vi "Swerve Drive Controller.vi"(8 "error in":errorcluster) -> ()   [LabVIEW 2015]
doc: "This VI executes continuously carrying out the current operation and responding to updates or new operations. It will often contain the timing or control code that is difficult to place directly in TeleOp. This VI generally opens all sensors and motors and isolates the rest of the robot code from knowing how the operations are carried out."
uses:
  Swerve Drive Setpoints.ctl
  Swerve Drive Operations.ctl
  <vilib>/Rock Robotics/WPI/CAN/TalonSRX/WPI_CANTalonSRX_APIControlMode.ctl
  Support Code/Team900-VIs/Team900SwerveDrive/SwerveDriveFuse.vi
  Swerve Drive Published Globals.vi
  <vilib>/Rock Robotics/Network Tables/SD Read Boolean.vi
  <vilib>/Rock Robotics/Network Tables/NT Read Numeric Array.vi
  Support Code/Team900-VIs/Team900SwerveDrive/SwerveGlobalData.vi
  Support Code/Team900-VIs/Team900SwerveDrive/Team900SwerveDrive.lvlib
  Support Code/Team900-VIs/navX Library v2/navX Library v2.lvlib
panel:
  out "Speed Chart":cluster{dbl, "Encoder Velocity":dbl}[](graph)
  out "Position Chart":cluster{dbl, "Encoder Velocity":dbl}[](graph)
  out "Current\nCmd":string
  # "Tip: It may be helpful to observe inputs and sensor values.\nYou may also want to display tuning or debugging controls."
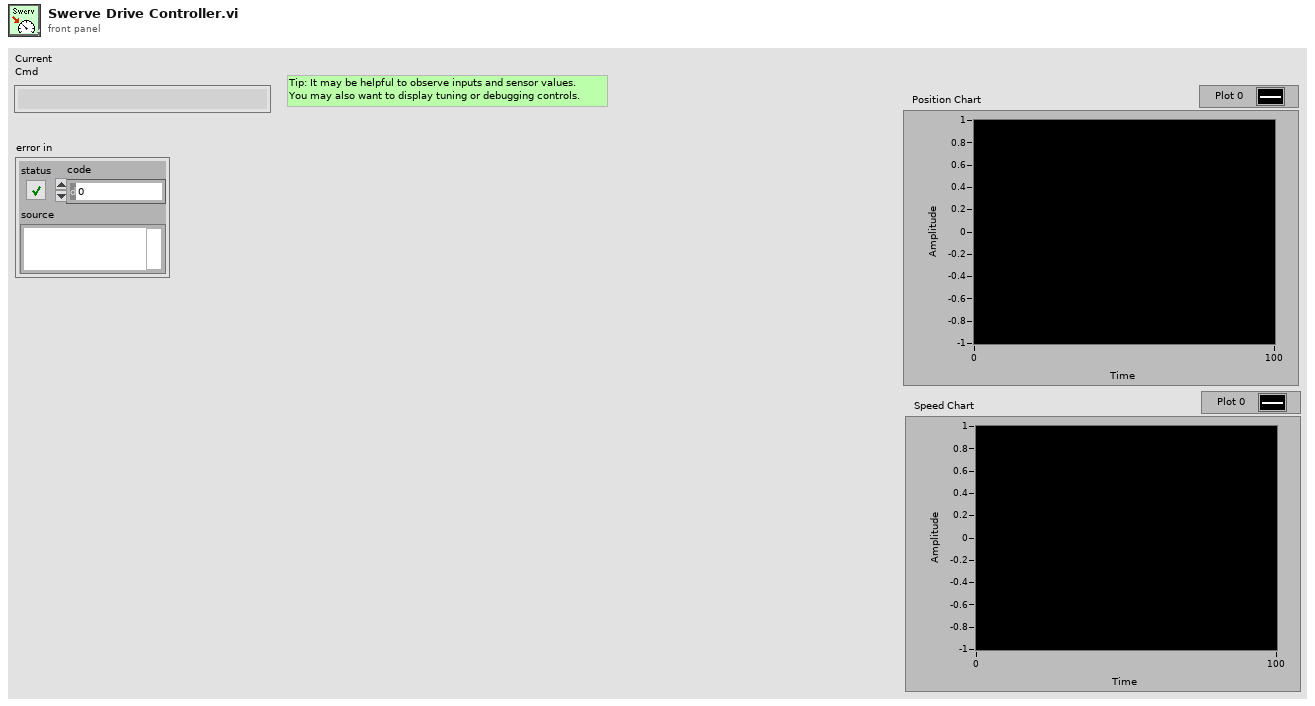
[diagram p1: front panel]
types:
  T1 = typedef "Swerve Drive Setpoints.ctl" = cluster{"Operation":T2, "Duration":dbl, "Strafe Joystick Axes":cluster{"X":dbl, "Y":dbl}, "Face Joystick Axes":cluster{"X":dbl, "Y":dbl}, "Trigger Axes":cluster{"Left":dbl, "Right":dbl}, "Coordinates":cluster{"X":dbl, "Y":dbl, "Angle":dbl}}
  T2 = typedef "Swerve Drive Operations.ctl" = enum16{"Reserve", "Read Current", "Immediate", "Go to Coordinate", "Drive Immediate (Turn Speed/Face and Stafe)"}
  T3 = typedef "Command Status Info.ctl" = cluster{"Name":string, "Status":T4, "notifier out":T5}
  T4 = typedef "Completion Status.ctl" = enum16{"Successful", "Aborted", "Incomplete"}
  T5 = typedef "Completion Notifier.ctl" = refnum<notifier>
  T6 = cluster{"Default Command":T1, "Command Timing":cluster{"Start Time (ms)":u32, "Iterations":i32}, "Command Arguments":cluster{"Command Info":T3, "Description":string, "Default Command":T1, "notifier out":refnum<notifier>, "Subsystem Name":string}}
  T7 = typedef "navX Library v2.lvlib/Z900_navX_DeviceTypeDef.ctl" = cluster{"Interface":cluster{"Protocol":T8, "Update Rate (4Hz-60Hz)":u8, "navX Open TypeDef":variant}, "Notify Packet":refnum<notifier>, "Loop VI Refnum":refnum<vi>, "Ready to Close Occurrence Refnum":refnum<k4>}
  T8 = typedef "navX Library v2.lvlib/Z900_navX_ProtocolTypeDef.ctl" = enum16{"SERIAL", "I2C", "SPI"}
  T9 = typedef "WPI_MotorControlDeviceRef.ctl" = cluster{"DeviceStatus":errorcluster, "Type":T10, "PWM":cluster{"PWM Channel":T11, "DeadBand":T12}, "CAN":cluster{"Device Number":u8, "Control Mode":T13, "Semaphore":T14, "Max Vout":dbl, "TalonSRX Control Mode":T15}, "Invert":bool}
  T10 = typedef "WPI_MotorControlType.ctl" = enum16{"PWM", "CAN", "CANTalonSRX"}
  T11 = typedef "FPGA_DIOPWMChannel.ctl" = enum8{"PWM 0", "PWM 1", "PWM 2", "PWM 3", "PWM 4", "PWM 5", "PWM 6", "PWM 7", "PWM 8", "PWM 9", "PWM MXP 0", "PWM MXP 1", "PWM MXP 2", "PWM MXP 3", "PWM MXP 4", "PWM MXP 5", "PWM MXP 6", "PWM MXP 7", "PWM MXP 8", "PWM MXP 9", "Invalid"}
  T12 = typedef "WPI_PWMDeadband.ctl" = cluster{"Name":string, "maxPositivePwm":i32, "minPositivePwm":i32, "centerPwm":i32, "maxNegativePwm":i32, "minNegativePwm":i32, "angularRange":u16}
  T13 = typedef "WPI_CANJaguar_ControlMode.ctl" = enum8{"Percent VBus", "Current", "Speed", "Position", "Voltage"}
  T14 = typedef "Semaphore RefNum" = refnum<k1>
  T15 = typedef "WPI_CANTalonSRX_APIControlMode.ctl" = enum8{"Percent VBus", "Speed", "Position", "Slave", "Unchanged / Invalid", "Voltage Compensation", "Current", "Motion Profile"}
  T16 = cluster{"Yaw":dbl, "Roll":dbl, "Pitch":dbl, "Heading":dbl, "Fused Heading":dbl}
  T17 = cluster{"Steering Motor Refs[0]":T9, "Steering Motor Refs[1]":T9, "Steering Motor Refs[2]":T9, "Steering Motor Refs[3]":T9}
  T18 = typedef "WPI_CANTalonSRX_GlobalStatus.ctl" = cluster{"Applied Throttle":dbl, "Module Enabled":bool, "CAN Error":errorcluster, "Closed Loop Error":dbl, "Forward Limit Switch Closed":bool, "Reverse Limit Switch Closed":bool, "Sensor Position":dbl, "Sensor Velocity":dbl, "Current":dbl, "Sticky Fault - Over Temp":bool, "Sticky Fault - Under Voltage":bool, "Sticky Fault - Forward Limit":bool, "Sticky Fault - Reverse Limit":bool, "Sticky Fault - Forward Soft Limit":bool, "Sticky Fault - Reverse Soft Limit":bool, "Brake is Enabled":bool, "Encoder Position":dbl, "Encoder Velocity":dbl, "Encoder Index Count":dbl, "Encoder A Pin State":bool, "Encoder B Pin State":bool, "Encoder Index Pin State":bool, "Analog In":dbl, "Analog In Velocity":dbl, "Temperature (C)":dbl, "Battery Voltage":dbl, "Control 5 Is Supported":bool, "Current Profile Slot Select":dbl, "Pos Div 8":bool, "Vel Div 4":bool, "Pulse Width Position":i32, "Pulse Width Velocity":i32, "Pulse Width Rise To Rise (us)":i32, "Pulse Width Rise To Fall (us)":i32, "Mot Prof Active Is Under Run":bool, "Mot Prof Active Has Under Run":bool, "Mot Prof Active Is Last":bool, "Mot Prof Active Velocity Only":bool, "Mot Prof Active Is Valid":bool, "Mot Prof Buffer Is Full":bool, "Mot Prof Active Profile Slot Select":i32, "Mot Prof NextID":i32, "Mot Prof Count":i32, "Mot Prof Active Velocity":dbl, "Mot Prof Active Position":dbl, "Mot Prof Output Enable":i32}
  T19 = cluster{"output angle":dbl, "Encoder Velocity":dbl}
  T20 = cluster{"[0]":dbl, "[1]":dbl, "[2]":dbl, "[3]":dbl}
  T21 = cluster{"Numeric Array[0]":dbl, "Numeric Array[1]":dbl, "Numeric Array[2]":dbl}
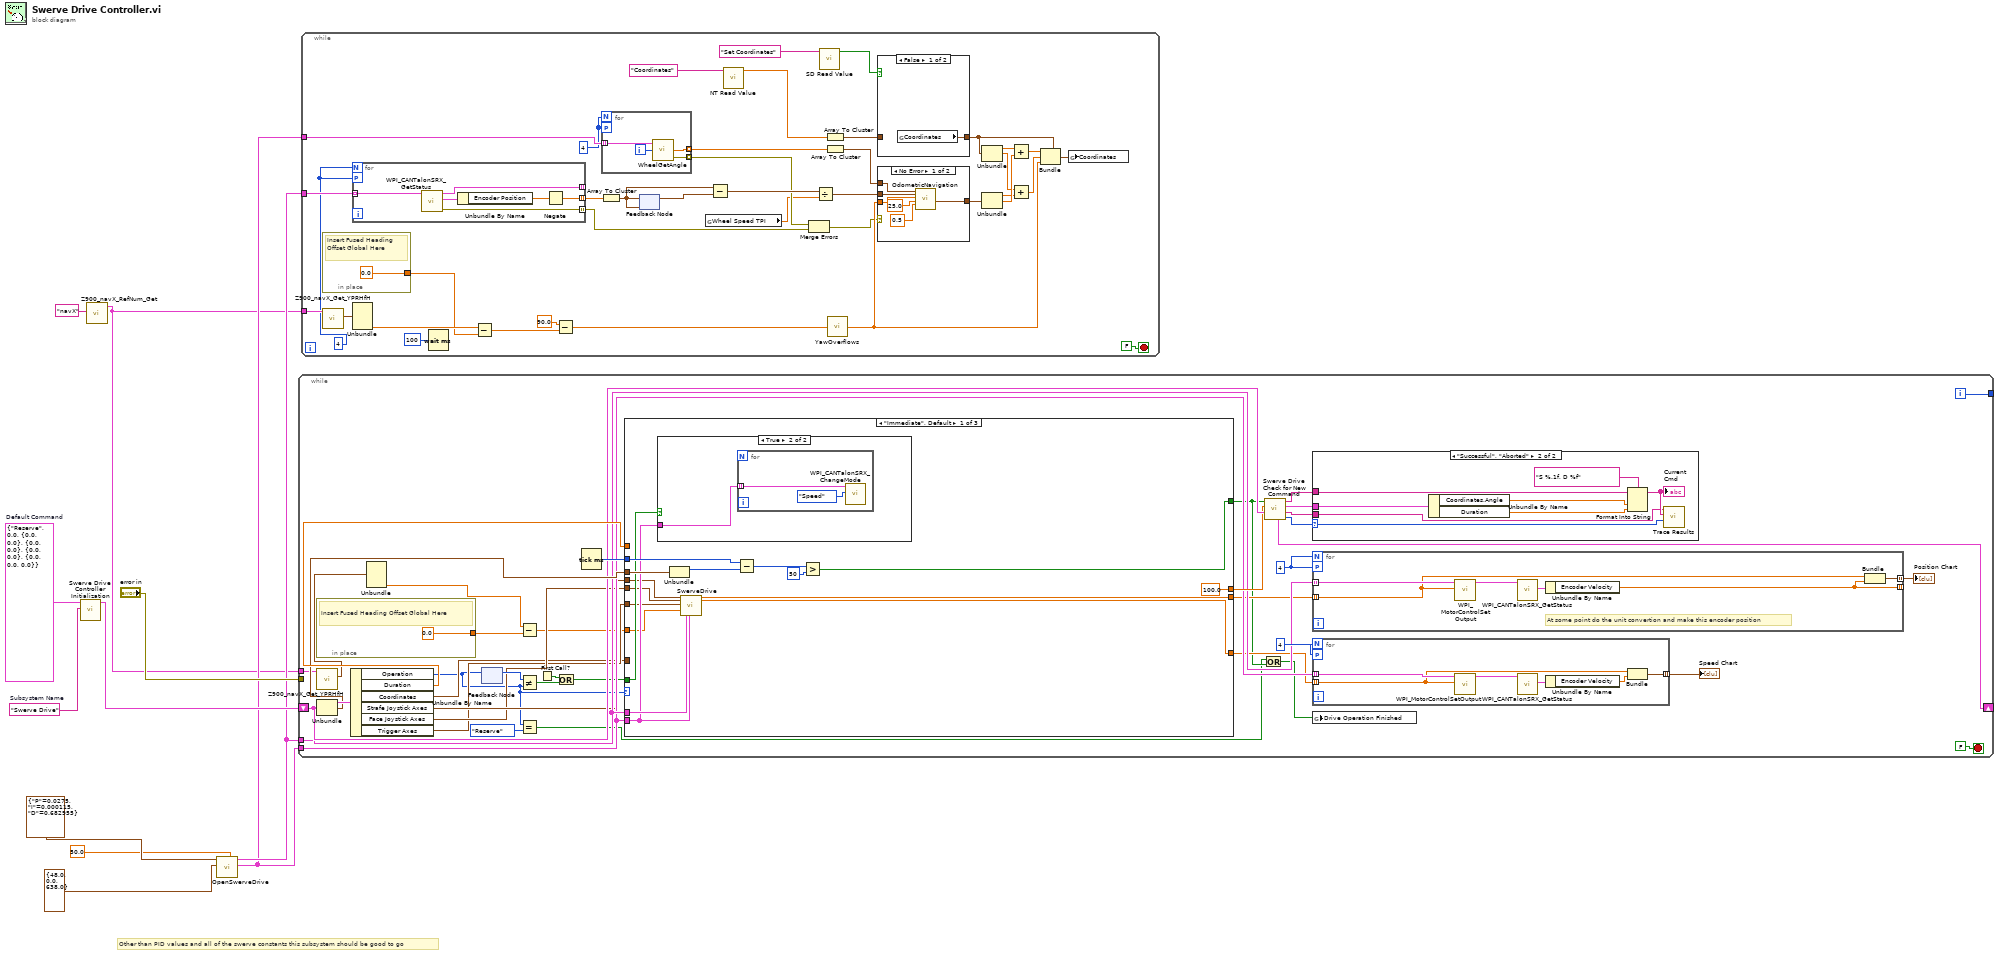
[diagram p0: block diagram]
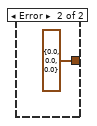
[diagram p2: hidden frame]
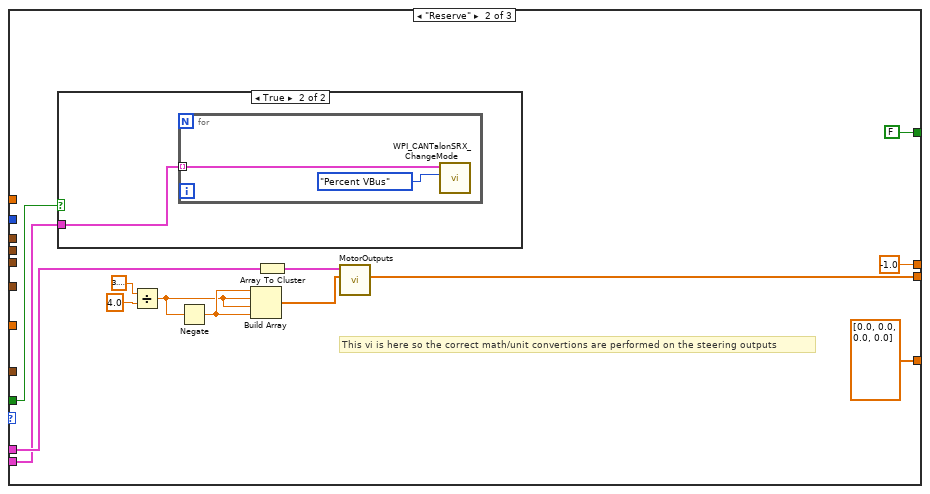
[diagram p6: hidden frame]
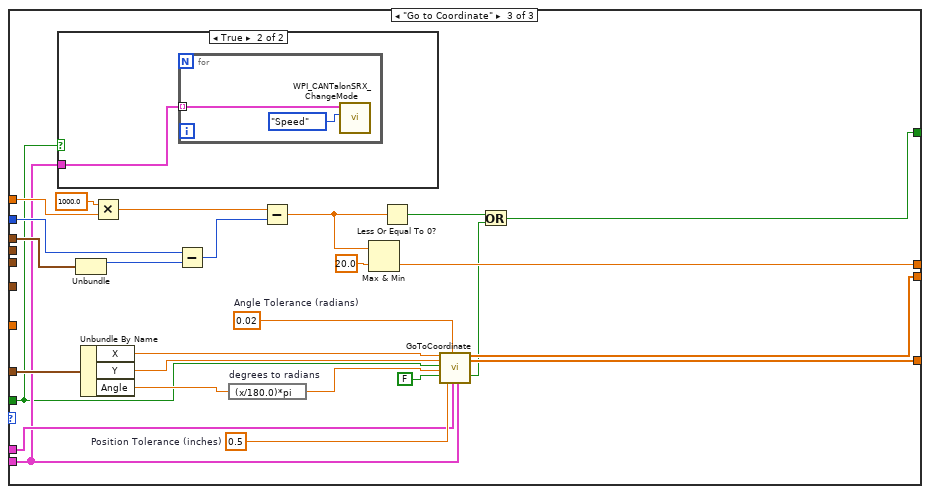
[diagram p8: hidden frame]
diagram:
  w8 = T1 {"Operation"=enum."Reserve", "Duration"=0.0, "Strafe Joystick Axes"={"X"=0.0, "Y"=0.0}, "Face Joystick Axes"={"X"=0.0, "Y"=0.0}, "Trigger Axes"={"Left"=0.0, "Right"=0.0}, "Coordinates"={"X"=0.0, "Y"=0.0, "Angle"=0.0}}  # Default Command
  w9 = "Swerve Drive"  # Subsystem Name
  # "Other than PID values and all of the swerve constants this subsystem should be good to go"
  n1 = call "Swerve Drive Controller Initialization.vi"("Subsystem Name"=w9, "Default Command"=w8) -> ("Command Info"=w10:T6)  [unwired: 9 in]
  n2 = call "Z900_navX_RefNum_Get.vi"("refnum name"="navX") -> ("navX Device"=w1:T7)  [unwired: 9 in, 1 out]
  n3 = call "OpenSwerveDrive.vi"("Ramp Rate"=50.0, "Speed PID"=cluster{"P":dbl, "I":dbl, "D":dbl} {"P"=48.0, "I"=0.0, "D"=638.0}, "Steering PID"=cluster{"P":dbl, "I":dbl, "D":dbl} {"P"=0.0275, "I"=0.000115, "D"=0.682955}) -> ("Speed Motor Refs"=w2:T9[], "Steering Motor Refs"=w3:T9[])  [unwired: 4 in, 1 out]
  n4 = while {
    shift-right: [w43] -> _
    shift-left: w10 -> [w44]
    tunnel: [w49] -> _
    tunnel: "error in" -> [_]
    tunnel: w3 -> [w33]
    tunnel: w2 -> [w32]
    tunnel: w1 -> [w13]
    i -> [w49]
    stop <- FALSE stop-if-true
    w34 = 4
    w35 = 4
    n5 = in-place {
      in-place-border: [0.0] -> w14
      # "Insert Fused Heading Offset Global Here"
    }
    n6 = call "Z900_navX_Get_YPRHfH.vi"("navX Device"=w13) -> ("YRPHfH"=w16:T16)  [unwired: 7 in, 3 out]
    n7 = Unbundle(w44) -> ("Default Command"=w48:T1, "Command Timing"=w45:cluster{"Start Time (ms)":u32, "Iterations":i32})  [unwired: 1 out]
    n8 = Unbundle By Name(w48) -> ("Operation"=w19:T2, "Duration"=w47:dbl, "Coordinates"=w22:cluster{"X":dbl, "Y":dbl, "Angle":dbl}, "Strafe Joystick Axes"=w25:cluster{"X":dbl, "Y":dbl}, "Face Joystick Axes"=w24:cluster{"X":dbl, "Y":dbl}, "Trigger Axes"=w23:cluster{"Left":dbl, "Right":dbl})
    n9 = Unbundle(w16) -> ("Fused Heading"=w15:dbl)  [unwired: 4 out]
    n10 = feedback-in #1(w19) -> ()
    n11 = feedback #1() -> (w29:T2)  [unwired: 1 in]
    n12 = Subtract(x=w15, y=w14) -> (x-y=w12:dbl)
    n13 = Not Equal?(x=w29, y=w19) -> (x != y?=w28:bool)
    n14 = Equal?(x=w19, y=Swerve_Drive_Operations."Reserve") -> (x = y?=w17:bool)
    n15 = First Call?() -> (First Call?: T/F=w27:bool)
    n16 = Or(x=w27, y=w28) -> (x .or. y?=w26:bool)
    n17 = Tick Count (ms)() -> (millisecond timer value=w46:u32)
    n18 = case shown="\"Immediate\", Default" w19 {
      tunnel: [100.0 -1.0 w121] -> w42
      tunnel: [w81 FALSE ("ignore previous (F)") w124] -> w21
      tunnel: w45 -> [w83 _ w132]
      tunnel: w47 -> [_ _ w129]
      tunnel: w46 -> [w82 _ w130]
      tunnel: w33 -> [w80 w94 w113]
      tunnel: w32 -> [w76 w91 w108]
      tunnel: [w79 w95 w111] -> w31
      tunnel: [w78 dbl[] [0.0, 0.0, 0.0, 0.0] ("appended array") w112] -> w30
      tunnel: w26 -> [w77 w92 w107]
      tunnel: w25 -> [w75 _ _]
      tunnel: w24 -> [w74 _ _]
      tunnel: w23 -> [w73 _ _]
      tunnel: w22 -> [_ _ w120]
      tunnel: w12 -> [w72 _ _]
      frame "Immediate", Default {
        n19 = case shown="True" w77 {
          tunnel: w76 -> [_ w88]
          frame False {
          }
          frame True {
            n20 = for {
              tunnel: w88 -> [w90] mode=indexing
              n21 = call <vilib>:"WPI_CANTalonSRX_ChangeMode.vi"("Control Mode"=WPI_CANTalonSRX_APIControlMode."Speed", "CAN Talon SRX Ref"=w90) -> ()  [unwired: 8 in, 2 out]
            }
          }
        }
        n22 = Unbundle(w83) -> ("Start Time (ms)"=w86:u32)  [unwired: 1 out]
        n23 = call-poly "SwerveDrive.vi"("Strafe Joystick Axes"=w75, "Face Joystick Axes"=w74, "Trigger Axes"=w73, "Angle (degrees; 0 = right)"=w72, "Steering Motor Refs"=w80, "Speed Motor Refs"=w76) -> ("Steering Motor Setpoints"=w79:dbl[], "Speed Motor Setpoints"=w78:dbl[])  [unwired: 10 in, 2 out]
        n24 = Subtract(x=w82, y=w86) -> (x-y=w85:u32)
        n25 = Greater?(x=w85, y=u8 50 ("Left Motor")) -> (0:w81:bool)
      }
      frame "Reserve" {
        # "This vi is here so the correct math/unit convertions are performed on the steering outputs"
        n26 = case shown="True" w92 {
          tunnel: w91 -> [_ w104]
          frame False {
          }
          frame True {
            n27 = for {
              tunnel: w104 -> [w106] mode=indexing
              n28 = call <vilib>:"WPI_CANTalonSRX_ChangeMode.vi"("Control Mode"=WPI_CANTalonSRX_APIControlMode."Percent VBus", "CAN Talon SRX Ref"=w106) -> ()  [unwired: 8 in, 2 out]
            }
          }
        }
        n29 = Divide(x=3.141592653589793, y=4.0) -> (x/y=w100:dbl)
        n30 = Negate(x=w100) -> (-x=w101:dbl)
        n31 = Build Array(w101, w100, w100, w101) -> (w97:dbl[])
        n32 = Array To Cluster(array=w94) -> (cluster=w93:T17)
        n33 = call "MotorOutputs.vi"("Target Angles"=w97, "Steering Refnums In"=w93) -> ("Steering Motor Setpoints"=w95:dbl[])  [unwired: 6 in, 3 out]
      }
      frame "Go to Coordinate" {
        w114 = 0.02  # Angle Tolerance (radians)
        w115 = 0.5  # Position Tolerance (inches)
        n34 = case shown="True" w107 {
          tunnel: w108 -> [_ w133]
          frame False {
          }
          frame True {
            n35 = for {
              tunnel: w133 -> [w135] mode=indexing
              n36 = call <vilib>:"WPI_CANTalonSRX_ChangeMode.vi"("Control Mode"=WPI_CANTalonSRX_APIControlMode."Speed", "CAN Talon SRX Ref"=w135) -> ()  [unwired: 8 in, 2 out]
            }
          }
        }
        n37 = Unbundle(w132) -> ("Start Time (ms)"=w131:u32)  [unwired: 1 out]
        n38 = Unbundle By Name(w120) -> ("X"=w119:dbl, "Y"=w118:dbl, "Angle"=w109:dbl)
        n39 = Multiply(x=1000.0, y=w129) -> (x*y=w127:dbl)
        n40 = Subtract(x=w130, y=w131) -> (x-y=w126:u32)
        n41 = expression code="(x/180.0)*pi" "degrees to radians"(w109) -> (w117:dbl)
        n42 = Subtract(x=w127, y=w126) -> (x-y=w123:dbl)
        n43 = Max & Min(x=w123, y=20.0) -> (min(x,y)=w121:dbl)  [unwired: 1 out]
        n44 = Less Or Equal To 0?(x=w123) -> (x <= 0?=w125:bool)
        n45 = call "GoToCoordinate.vi"("Target X"=w119, "Target Y"=w118, "Reset (for robot centric)"=w107, "Target Angle (rad)"=w117, "Field Centric?"=FALSE, "Position Tolerance"=w115, "Angle Tolerance"=w114, "Steering Motor Refs"=w113, "Speed Motor Refs"=w108) -> ("Steering Motor Setpoints"=w111:dbl[], "Speed Motor Setpoints"=w112:dbl[], "Finished"=w110:bool)  [unwired: 7 in, 1 out]
        n46 = Or(x=w125, y=w110) -> (x .or. y?=w124:bool)
      }
    }
    n47 = Or(x=w17, y=w21) -> (x .or. y?=w20:bool)
    n48 = call "Swerve Drive Check for New Command.vi"("Current Command"=w44, "Wait time (ms)"=w42, "Finished?"=w21) -> ("Completion"=w38:T4, "Subsystem Name"=w39:string, "Current Command"=w40:T1, "Initial Trace String"=w41:string, "NextCommand"=w43:T6)  [unwired: 4 in]
    n49 = case shown="\"Successful\", \"Aborted\"" w38 {
      selector: w38 -> [_ w71]
      tunnel: w41 -> [_ w67]
      tunnel: w40 -> [_ w68]
      tunnel: w39 -> [_ w64]
      frame "Incomplete", Default {
        # "Continuing current command"
      }
      frame "Successful", "Aborted" {
        # "Report and setup for next command"
        n50 = Unbundle By Name(w68) -> ("Coordinates.Angle"=w70:dbl, "Duration"=w65:dbl)
        n51 = Format Into String(format string="S %.1f, D %f", initial string=w67, w70, w65) -> (resulting string=w66:string)  [unwired: 1 in, 1 out]
        "Current\nCmd" <- w66
        n52 = call <vilib>:"Trace Results.vi"("Status of previous command"=w71, "Description"=w66, "Subsystem"=w64) -> ()  [unwired: 9 in]
      }
    }
    n53 = for {
      N: w34 -> [_]
      workers-P: w34 -> [_]
      tunnel: w33 -> [w63] mode=indexing
      tunnel: [w61] -> _ mode=indexing
      tunnel: [w60] -> w37 mode=indexing
      tunnel: w31 -> [w59] mode=indexing
      # "At some point do the unit convertion and make this encoder position"
      n54 = call <vilib>:"WPI_MotorControlSetOutput.vi"("Output"=w59, "MotorControlDevRef"=w63) -> ("MotorControlDevRef"=w62:T9)  [unwired: 7 in, 2 out]
      n55 = call <vilib>:"WPI_CANTalonSRX_GetStatus.vi"("CAN Talon SRX Ref"=w62) -> ("Talon SRX Status"=w58:T18)  [unwired: 8 in, 2 out]
      n56 = Unbundle By Name(w58) -> ("Encoder Velocity"=w61:dbl)
      n57 = Bundle("output angle"=w59, "Encoder Velocity"=w61) -> (w60:T19)  [unwired: 1 in]
    }
    "Position Chart" <- w37
    n58 = for {
      N: w35 -> [_]
      workers-P: w35 -> [_]
      tunnel: w32 -> [w57] mode=indexing
      tunnel: w30 -> [w53] mode=indexing
      tunnel: [w52] -> w36 mode=indexing
      n59 = call <vilib>:"WPI_MotorControlSetOutput.vi"("Output"=w53, "MotorControlDevRef"=w57) -> ("MotorControlDevRef"=w55:T9)  [unwired: 7 in, 2 out]
      n60 = call <vilib>:"WPI_CANTalonSRX_GetStatus.vi"("CAN Talon SRX Ref"=w55) -> ("Talon SRX Status"=w56:T18)  [unwired: 8 in, 2 out]
      n61 = Unbundle By Name(w56) -> ("Encoder Velocity"=w54:dbl)
      n62 = Bundle(w53, "Encoder Velocity"=w54) -> (w52:cluster{dbl, "Encoder Velocity":dbl})  [unwired: 1 in]
    }
    "Speed Chart" <- w36
    n63 = global write "Swerve Drive Published Globals.vi" "Drive Operation Finished"(w20) -> ()
  }
  n64 = while {
    tunnel: w1 -> [w173]
    tunnel: w3 -> [w171]
    tunnel: w2 -> [w170]
    stop <- FALSE stop-if-true
    w144 = 4
    w145 = 4
    n65 = in-place {
      in-place-border: [0.0] -> w167
      # "Insert Fused Heading Offset Global Here"
    }
    n66 = call "Z900_navX_Get_YPRHfH.vi"("navX Device"=w173) -> ("YRPHfH"=w169:T16)  [unwired: 7 in, 3 out]
    n67 = for {
      N: w145 -> [_]
      tunnel: [w189] -> _ mode=indexing
      tunnel: [w191] -> w155 mode=indexing
      workers-P: w145 -> [_]
      tunnel: w171 -> [w188] mode=indexing
      tunnel: [w187] -> w149 mode=indexing
      n68 = call <vilib>:"WPI_CANTalonSRX_GetStatus.vi"("CAN Talon SRX Ref"=w188) -> ("error out"=w191:errorcluster, "Talon SRX Status"=w190:T18, "CAN Talon SRX Ref"=w189:T9)  [unwired: 8 in]
      n69 = Unbundle By Name(w190) -> ("Encoder Position"=w186:dbl)
      n70 = Negate(x=w186) -> (-x=w187:dbl)
    }
    n71 = Unbundle(w169) -> ("Fused Heading"=w168:dbl)  [unwired: 4 out]
    n72 = Wait (ms)(milliseconds to wait=u32 100) -> ()  [unwired: 1 out]
    n73 = Subtract(x=w168, y=w167) -> (x-y=w139:dbl)
    n74 = Subtract(x=90.0, y=w139) -> (x-y=w161:dbl)
    n75 = Array To Cluster(array=w149) -> (cluster=w150:T20)
    n76 = for {
      N: w144 -> [_]
      workers-P: w144 -> [_]
      tunnel: [w177] -> w148 mode=indexing
      tunnel: w170 -> [w176] mode=indexing
      tunnel: [w175] -> w146 mode=indexing
      i -> [w178]
      n77 = call "WheelGetAngle.vi"("Wheel"=w178, "CAN Talon SRX Ref"=w176) -> ("error out"=w177:errorcluster, "Sensor Position (rad)"=w175:dbl)  [unwired: 1 in, 1 out]
    }
    n78 = feedback #2(w150) -> (w151:T20)
    n79 = feedback-in #2(w150) -> ()
    n80 = global read "SwerveGlobalData.vi" "Wheel Speed TPI"() -> (w137:dbl)
    n81 = Subtract(x=w150, y=w151) -> (x-y=w152:T20)
    n82 = call-poly <vilib>:"NT Read Value.vi"("Name"="Coordinates") -> ("Numeric Array"=w143:dbl[])  [unwired: 9 in, 1 out]
    n83 = Merge Errors(w148, w155) -> (w154:errorcluster)
    n84 = Divide(x=w152, y=w137) -> (x/y=w153:T20)
    n85 = call-poly <vilib>:"SD Read Value.vi"("Name"="Set Coordinates") -> ("Boolean"=w140:bool)  [unwired: 8 in, 2 out]
    n86 = Array To Cluster(array=w143) -> (cluster=w142:T21)
    n87 = Array To Cluster(array=w146) -> (cluster=w147:T20)
    n88 = call "YawOverflows.vi"("Yaw (degrees)"=w161) -> ("Yaw (with overflows)"=w163:dbl)
    n89 = case shown="False" w140 {
      tunnel: [w192 w193] -> w166
      tunnel: w142 -> [_ w193]
      frame False {
        n90 = global read "SwerveGlobalData.vi" "Coordinates"() -> (w192:cluster{"X":dbl, "Y":dbl, "Heading":dbl})
      }
      frame True {
      }
    }
    n91 = case shown="No Error" w154 {
      tunnel: [w182 cluster{"sy":dbl, "sx":dbl, "rot.":dbl} {"sy"=0.0, "sx"=0.0, "rot."=0.0} ("movement")] -> w156
      tunnel: w153 -> [w184 _]
      tunnel: w147 -> [w183 _]
      tunnel: w163 -> [w179 _]
      frame No Error {
        n92 = call "OdometricNavigation.vi"("Wheel Angles (rad)"=w183, "Wheel Movements (in.)"=w184, "Robot angle (degrees)"=w179, "x and y error minimum (in.)"=25.0, "error minimum for rotation (rad)"=0.5 ("error minimum for rotation (in.)")) -> ("movement"=w182:cluster{"sy":dbl, "sx":dbl, "rot.":dbl})  [unwired: 14 in]
      }
      frame Error {
      }
    }
    n93 = Unbundle(w166) -> ("Numeric Array[0]"=w160:dbl, "Numeric Array[1]"=w158:dbl)  [unwired: 1 out]
    n94 = Unbundle(w156) -> ("sy"=w157:dbl, "sx"=w159:dbl)  [unwired: 1 out]
    n95 = Add(x=w160, y=w159) -> (x+y=w165:dbl)
    n96 = Add(x=w158, y=w157) -> (x+y=w164:dbl)
    n97 = Bundle(cluster=w166, "Numeric Array[0]"=w165, "Numeric Array[1]"=w164, "Numeric Array[2]"=w163) -> (w136:T21)
    n98 = global write "SwerveGlobalData.vi" "Coordinates"(w136) -> ()
  }
